vi "Create.vi"(8 "error in (no error)":errorcluster, 9 "Red Threshold":dbl, 10 "Green Threshold":dbl) -> (0 "error out":errorcluster, 3 "Aim Lower Threshold out":refnum<class "Aim Lower Threshold.lvclass">)   [LabVIEW 2021, in "Aim Lower Threshold.lvclass"]
uses:
  Aim Lower Threshold.lvclass
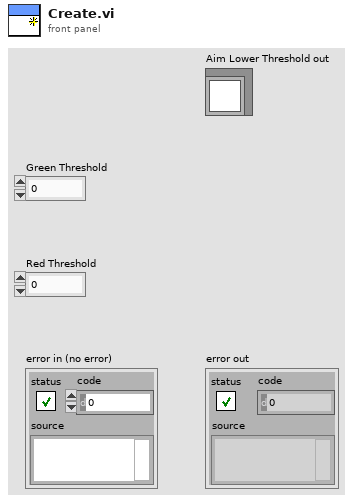
[diagram p1: front panel]
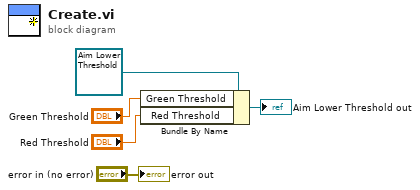
[diagram p0: block diagram]
diagram:
  n1 = Bundle By Name(cluster=refnum<class "Aim Lower Threshold.lvclass"> refnum ("Aim Lower Threshold in"), "Green Threshold"="Green Threshold", "Red Threshold"="Red Threshold") -> (→"Aim Lower Threshold out":refnum<class "Aim Lower Threshold.lvclass">)
  "error out" <- "error in (no error)"
